vi "recv_pck_str.vi"(11 "inp_pck":T1) -> (3 "res_str":string)   [LabVIEW 2021]
uses:
  typedefs/w5500_pck.ctl
  typedefs/w5500_cmd.ctl
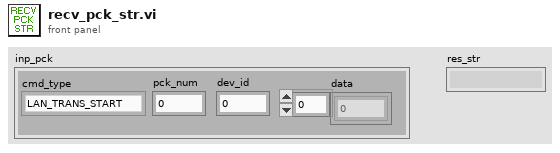
[diagram p1: front panel]
types:
  T1 = typedef "w5500_pck.ctl" = cluster{"cmd_type":T2, "pck_num":u32, "dev_id":u32, "data":u8[]}
  T2 = typedef "w5500_cmd.ctl" = enum32{"LAN_TRANS_START", "LAN_DATA_SZ", "LAN_CHUNK_SEND", "LAN_CHUNK_ACK", "LAN_DEVS_INFO", "LAN_DEVS_NUM", "LAN_DEVS_EXS", "LAN_DEVS_ACK", "LAN_CMD_ACK", "LAN_CMD_FIN", "LAN_SND_STAT", "LAN_REQ_STAT", "LAN_ANS_STAT", "LAN_ERR_STAT", "LAN_SETT_SET", "LAN_SETT_GET", "LAN_SETT_ACK", "LAN_SETT_ERR"}
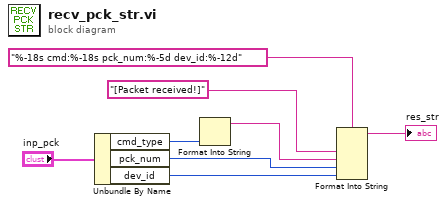
[diagram p0: block diagram]
diagram:
  n1 = Unbundle By Name("inp_pck") -> ("cmd_type"=w8:T2, "pck_num"=w4:u32, "dev_id"=w3:u32)
  n2 = Format Into String(w8) -> (resulting string=w5:string)  [unwired: 3 in, 1 out]
  n3 = Format Into String(format string="%-18s cmd:%-18s pck_num:%-5d dev_id:%-12d", "[Packet received!]", w5, w4, w3) -> (resulting string=→"res_str":string)  [unwired: 2 in, 1 out]
